vi "Auto InTake.vi"(3 "Auto InTake?":bool, 4 "Kick Info":T2, 5 "Intake Info In":T1) -> (0 "Lower Claw":dbl, 1 "Upper Claw":dbl, 2 "TakeBall":dbl)   [LabVIEW 2013]
panel:
  in  "error in (no error)":errorcluster
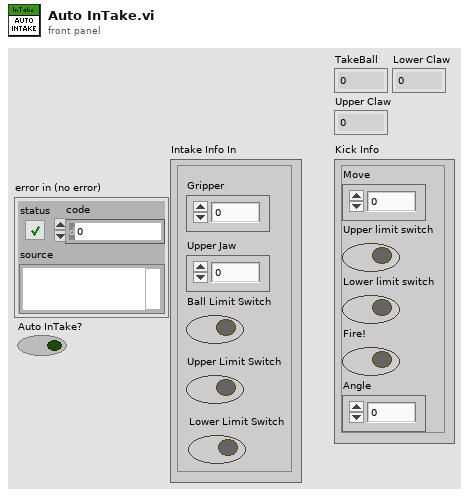
[diagram p1: front panel]
types:
  T1 = cluster{"Gripper":dbl, "Upper Jaw":dbl, "Ball Limit Switch":bool, "Upper Limit Switch":bool, "Lower Limit Switch ":bool}
  T2 = cluster{"Move":dbl, "Upper limit switch":bool, "Lower limit switch ":bool, "Fire!":bool, "Angle":dbl}
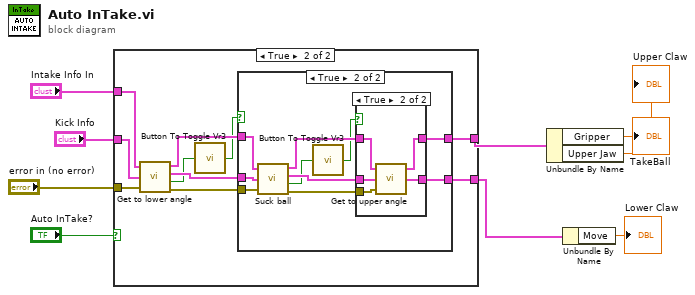
[diagram p0: block diagram]
diagram:
  n1 = case shown="True" "Auto InTake?" {
    tunnel: "error in (no error)" -> [_ w20]
    tunnel: "Kick Info" -> [w10 w18]
    tunnel: "Intake Info In" -> [w11 w16]
    tunnel: [w11 w14] -> w5
    tunnel: [w10 w15] -> w4
    frame False {
    }
    frame True {
      n2 = call "Get to lower angle.vi"("Intake Info In"=w16, "Kick Info"=w18, "error in (no error)"=w20) -> ("Intake Info Out"=w17:T1, "Kick Info"=w19:T2, "Finished"=w13:bool, "error out"=w21:errorcluster)
      n3 = call "Button To Toggle Vr3.vi"("InValue"=w13) -> ("Result"=w12:bool)
      n4 = case shown="True" w12 {
        tunnel: w21 -> [_ w32]
        tunnel: w19 -> [w22 w31]
        tunnel: w17 -> [w23 w29]
        tunnel: [w22 w28] -> w15
        tunnel: [w23 w26] -> w14
        frame False {
        }
        frame True {
          n5 = call "Suck ball.vi"("Intake Info In"=w29, "Kick Info"=w31, "error in (no error)"=w32) -> ("Intake Info Out"=w27:T1, "Kick Info"=w30:T2, "Finished?"=w24:bool, "error out"=w33:errorcluster)
          n6 = call "Button To Toggle Vr3.vi"("InValue"=w24) -> ("Result"=w25:bool)
          n7 = case shown="True" w25 {
            tunnel: w33 -> [_ w40]
            tunnel: w30 -> [w34 w39]
            tunnel: [w34 w38] -> w28
            tunnel: w27 -> [w35 w37]
            tunnel: [w35 w36] -> w26
            frame False {
            }
            frame True {
              n8 = call "Get to upper angle.vi"("error in (no error)"=w40, "Kick Info"=w39, "Intake Info In"=w37) -> ("Kick Info"=w38:T2, "Intake Info Out"=w36:T1)  [unwired: 1 out]
            }
          }
        }
      }
    }
  }
  n9 = Unbundle By Name(w5) -> ("Gripper"=→"TakeBall":dbl, "Upper Jaw"=→"Upper Claw":dbl)
  n10 = Unbundle By Name(w4) -> ("Move"=→"Lower Claw":dbl)
